vi "Day 18-Addition.vi"(10 "Data 2 in":i32[][](array[numeric]), 11 "Data 1 in":i32[][](array[numeric])) -> (3 "Data out":i32[][](array[numeric]))   [LabVIEW 2021]
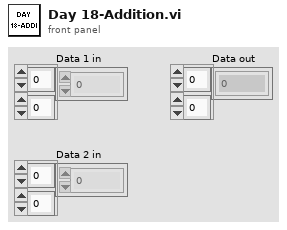
[diagram p1: front panel]
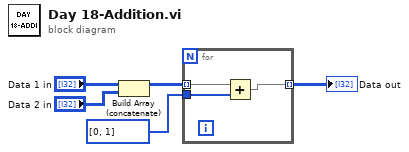
[diagram p0: block diagram]
diagram:
  n1 = Build Array (concatenate)("Data 1 in", "Data 2 in") -> (w2:i32[][])
  n2 = for {
    tunnel: w2 -> [w8] mode=indexing
    tunnel: i32[] [0, 1] -> [w7]
    tunnel: [w6] -> w4 mode=indexing
    n3 = Add(x=w8, y=w7) -> (x+y=w6:i32[])
  }
  "Data out" <- w4
